vi "Read.vi"(11 "Logger Status Value in":refnum<class "Logger Status Value.lvclass">) -> (2 "Logger Status":T1)   [LabVIEW 2020, in "VolatusHistorian.lvlib" / "Logger Status Value.lvclass"]
uses:
  Logger Status Value.lvclass
  Logger Status Value.lvclass/Logger Status Value.ctl
  Logger Status.ctl
  VolatusHistorian.lvlib
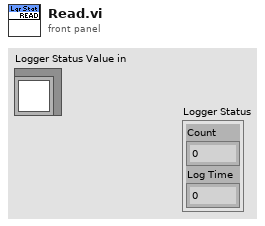
[diagram p1: front panel]
types:
  T1 = typedef "VolatusHistorian.lvlib/Logger Status.ctl" = cluster{"Count":i32, "Log Time":dbl}
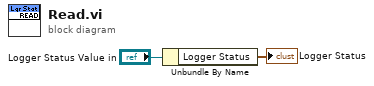
[diagram p0: block diagram]
diagram:
  n1 = Unbundle By Name("Logger Status Value in") -> ("Logger Status"=→"Logger Status":T1)
